vi "Set Control Level.vi"(6 "Mouse Position":T1, 7 "User VI Ref":refnum<vi>, 8 "Is Multi-select?":bool, 9 "Remaining Items":refnum<vi>[](array[refnum]), 10 "Affected Items":T8, 11 "Menu Refnum":refnum<k9>) -> (3 "Menu Items To Add":T2[](array[typedef]))   [LabVIEW 2021]
doc: "This implementation of the right click menu VI will set the \"UI Theme Level\" for a given control(s) for a VI. It will categorize the type of the control style that is being used so that Theme-ing can be applied appropriately.\n\n<b>Original</b>: This VI is part of a plug-in for modifying the LabVIEW shortcut menus. This is the builder VI which is called when the shortcut menu is built. It tells LabVIEW which shortcut menu items to add to the menu."
uses:
  <resource>/plugins/PopupMenus/support/Shortcut Menu Item Definition.ctl
  <resource>/plugins/PopupMenus/support/Transaction Control.ctl
  <resource>/plugins/PopupMenus/support/Position In Menu.ctl
  <resource>/plugins/PopupMenus/support/Relative Position.ctl
  <resource>/plugins/PopupMenus/support/Checkmark Status.ctl
  <resource>/plugins/PopupMenus/support/Enabled Menu Item Status.ctl
  Set Control Level.ctl
  <vilib>/Utility/miscctls.llb/LVPositionTypeDef.ctl
  4ff4612b-3443-4282-827c-392bf86662e1.vi
  Material SubVIs/Material SubVIs.lvlib
panel:
  # "Rules a popup plug-in must follow:\n* This VI's file name must match the file name of the LLB -- only the file extensions should be different.\n* This VI must have debugging disabled or it will be ignored as a plug-in.\n* For all menu items, \"tag suffix + file name of this VI\" must be less than 240 characters.\n* You can disconnect the \"Affected Items\" from the typedef to make the plug-in load faster. The typedef is only there to assist you in keeping this VI and the execution VI using to the same type.\n* All controls on this panel except \"Affected Items\" are locked to prevent accidental edits. Do not change the types or the names of controls other than the elements inside the \"Affected Items\" cluster.\n* See Context Help for more information on the individual controls."
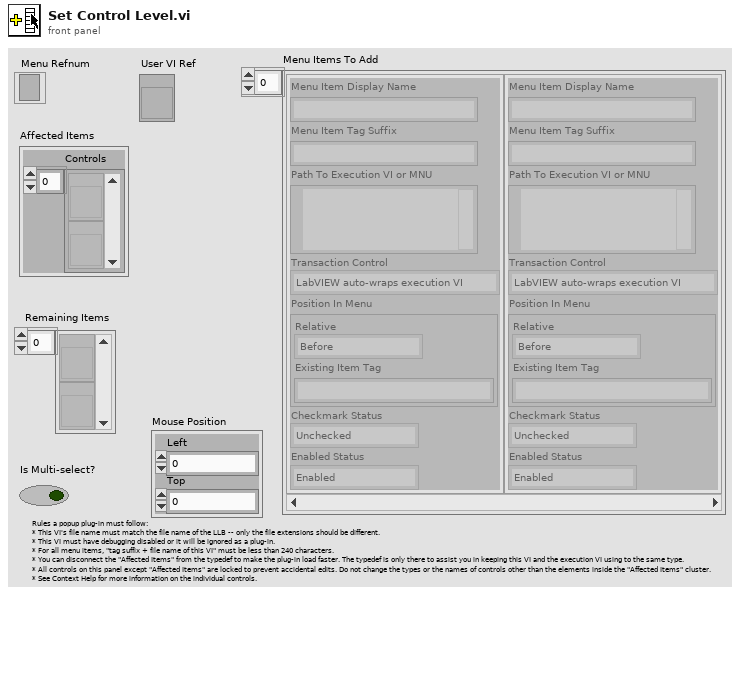
[diagram p1: front panel]
types:
  T1 = typedef "LVPositionTypeDef.ctl" = cluster{"Left":i32, "Top":i32}
  T2 = typedef "Shortcut Menu Item Definition.ctl" = cluster{"Menu Item Display Name":string, "Menu Item Tag Suffix":string, "Path To Execution VI or MNU":path, "Transaction Control":T3, "Position In Menu":T4, "Checkmark Status":T6, "Enabled Status":T7}
  T3 = typedef "Transaction Control.ctl" = enum8{"LabVIEW auto-wraps execution VI", "Execution VI will define if needed"}
  T4 = typedef "Position In Menu.ctl" = cluster{"Relative":T5, "Existing Item Tag":string}
  T5 = typedef "Relative Position.ctl" = enum8{"Before", "Instead of", "After", "Into Submenu"}
  T6 = typedef "Checkmark Status.ctl" = enum8{"Unchecked", "Checked"}
  T7 = typedef "Enabled Menu Item Status.ctl" = enum8{"Enabled", "Disabled"}
  T8 = typedef "Set Control Level.ctl" = cluster{"Controls":refnum<vi>[]}
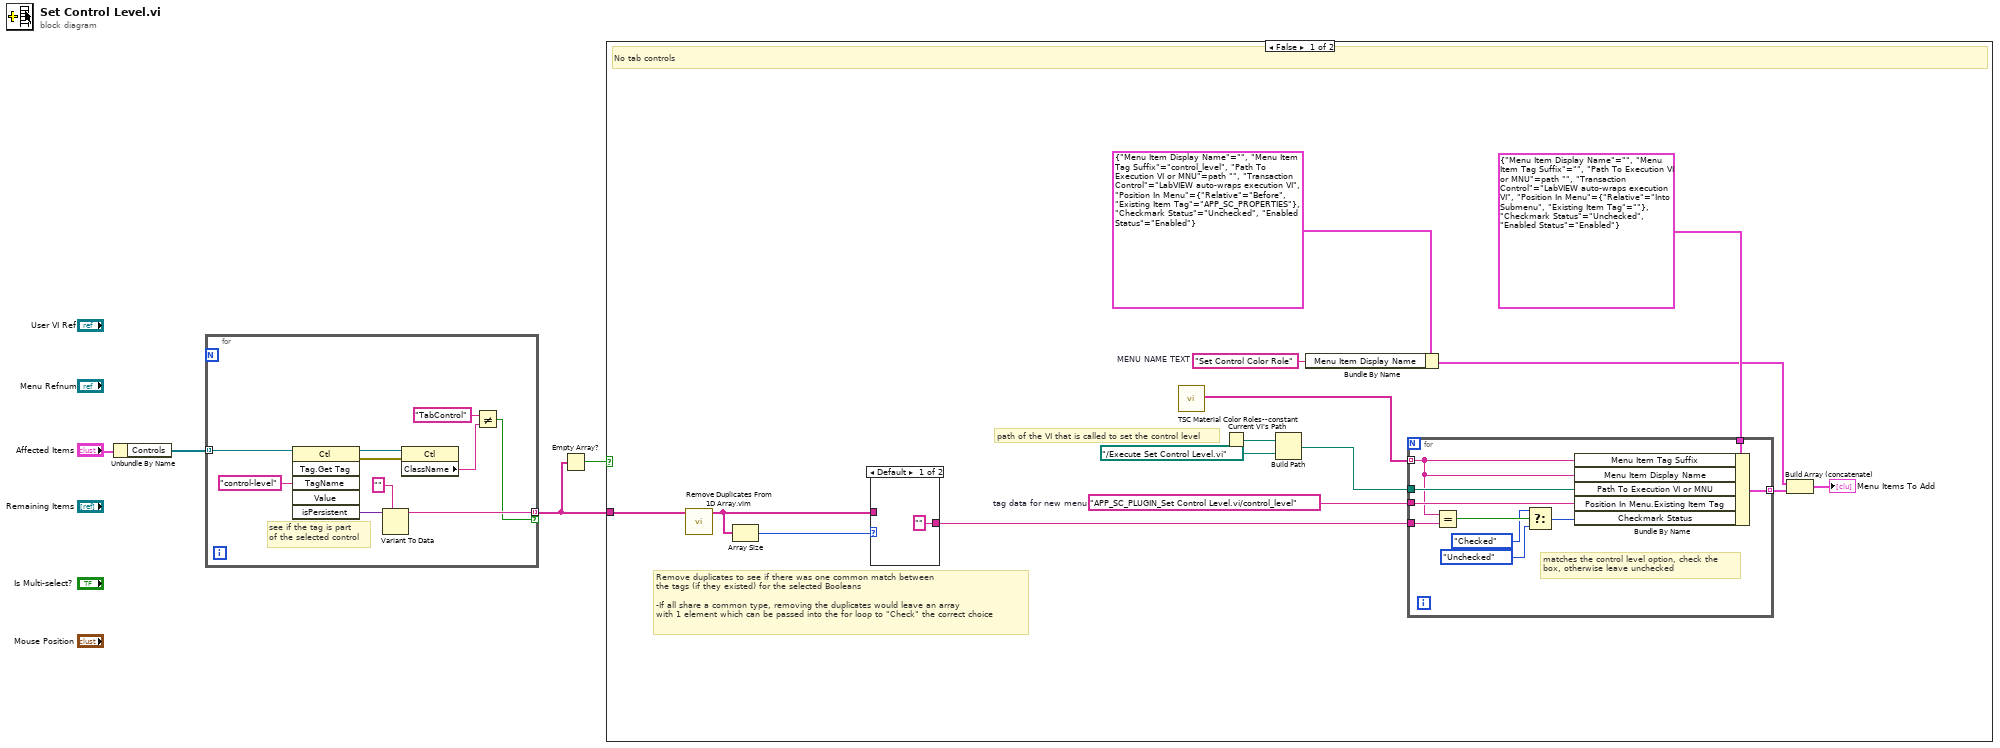
[diagram p0: block diagram]
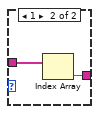
[diagram p2: hidden frame]
diagram:
  n1 = Unbundle By Name("Affected Items") -> ("Controls"=w3:refnum<vi>[])
  n2 = for {
    tunnel: w3 -> [w10] mode=indexing
    tunnel: [w11] -> w2 mode=indexing if=w5
    # "see if the tag is part \nof the selected control"
    n3 = invoke class="Ctl" method="Tag.Get Tag"(reference=w10, "TagName"="control-level" ("Tag Name")) -> (reference out=w8:refnum<vi>, error out=w9:errorcluster, "isPersistent"=w13:variant)  [unwired: 4 in, 3 out]
    n4 = Variant To Data(type="", Variant=w13) -> (data=w11:string)  [unwired: 1 in, 1 out]
    n5 = property class="Ctl"(reference=w8, error in=w9) -> ("ClassName"=w7:string)  [unwired: 2 out]
    n6 = Not Equal?(x="TabControl", y=w7) -> (x != y?=w5:bool)
  }
  n7 = Empty Array?(array=w2) -> (empty?=w1:bool)
  n8 = case shown="False" w1 {
    tunnel: w2 -> [w22 _]
    frame False {
      w15 = "APP_SC_PLUGIN_Set Control Level.vi/control_level"  # tag data for new menu
      w18 = "Set Control Color Role"  # MENU NAME TEXT
      # "Remove duplicates to see if there was one common match between\nthe tags (if they existed) for the selected Booleans\n\n-If all share a common type, removing the duplicates would leave an array\nwith 1 element which can be passed into the for loop to \"Check\" the correct choice"
      # "path of the VI that is called to set the control level"
      # "No tab controls"
      n9 = call "Remove Duplicates From 1D Array.vim"("array"=w22) -> ("array with duplicates removed"=w23:string[])  [unwired: 10 in]
      n10 = Array Size(array=w23) -> (size(s)=w24:i32)
      n11 = case shown="Default" w24 {
        tunnel: w23 -> [_ w32]
        tunnel: ["" w31] -> w21
        frame Default {
        }
        frame 1 {
          n12 = Index Array(array=w32) -> (element=w31:string)  [unwired: 1 in]
        }
      }
      n13 = call "TSC Material Color Roles--constant.vi"() -> ("Control Color Roles"=w20:string[])  [unwired: 11 in]
      n14 = Current VI's Path() -> (path=w28:path)
      n15 = Build Path(base path=w28, name or relative path=path "../Execute Set Control Level.vi" ("execute path")) -> (appended path=w27:path)
      n16 = Bundle By Name(cluster=T2 {"Menu Item Display Name"="", "Menu Item Tag Suffix"="control_level", "Path To Execution VI or MNU"=path "", "Transaction Control"=enum."LabVIEW auto-wraps execution VI", "Position In Menu"={"Relative"=enum."Before", "Existing Item Tag"="APP_SC_PROPERTIES"}, "Checkmark Status"=enum."Unchecked", "Enabled Status"=enum."Enabled"} ("Cluster"), "Menu Item Display Name"=w18) -> (w16:T2)
      n17 = for {
        tunnel: T2 {"Menu Item Display Name"="", "Menu Item Tag Suffix"="", "Path To Execution VI or MNU"=path "", "Transaction Control"=enum."LabVIEW auto-wraps execution VI", "Position In Menu"={"Relative"=enum."Into Submenu", "Existing Item Tag"=""}, "Checkmark Status"=enum."Unchecked", "Enabled Status"=enum."Enabled"} ("Cluster") -> [w42]
        tunnel: [w41] -> w26 mode=indexing
        tunnel: w27 -> [w40]
        tunnel: w15 -> [w39]
        tunnel: w20 -> [w33] mode=indexing
        tunnel: w21 -> [w35]
        # "matches the control level option, check the \nbox, otherwise leave unchecked"
        n18 = Equal?(x=w33, y=w35) -> (x = y?=w38:bool)
        n19 = Select(t=Checkmark_Status."Checked" ("Checkmark Status"), s=w38, f=Checkmark_Status."Unchecked" ("Checkmark Status")) -> (s? t:f=w34:T6)
        n20 = Bundle By Name(cluster=w42, "Menu Item Tag Suffix"=w33, "Menu Item Display Name"=w33, "Path To Execution VI or MNU"=w40, "Position In Menu.Existing Item Tag"=w39, "Checkmark Status"=w34) -> (w41:T2)
      }
      n21 = Build Array (concatenate)(w16, w26) -> (→"Menu Items To Add":T2[])
    }
    frame True {
      # "if any are tab controls, don't show"
    }
  }
